vi "Convert_to_2009.vi"(8 "error in (no error)":errorcluster, 10 "2009 data in":T1={"DistSettings"={"BuildLabel"="", "ProductName"="", "BuildLocation"=path "", "MediaSize"=0, "Language"=9, "ProductVersion"={"Major"=1, "Minor"=0, "Update"=0}, "AutoIncrement"=FALSE, "ReadmeID"="", "LicenseID"="", "arpCompany"="", "arpURL"="http://", "arpContact"="", "arpPhone"="", "Executable"="", "CmdArg"="", "OSCheck"=0, "Hide"=FALSE, "LV80higher"=FALSE, "IncludeError?"=FALSE, "HWOption"=enum."<none>", "HWPath"=path "", "UpgradeCode"="", "Author"="", "MsiFileName"="", "CabFileName"="", "DistID"="", "WindowTitle"="", "WindowMessage"="", "CacheDistros"=FALSE, "EXE str ref?"=FALSE}, "BldInfo"=[], "FileInfo"=[], "DirInfo"=[], "ShortcutInfo"=[], "RegInfo"=[], "RegData"=[], "DistParts"=[], "DefaultDir"=""} {"RegData"."Values"."Type" items=["Bare", "String", "Expandable String", "Binary", "DWord"]; "DistSettings"."ProductVersion"."Update" step=1; "DistSettings"."ProductVersion"."Minor" step=1; "DistSettings"."ProductVersion"."Major" step=1; "DistSettings"."Language" items=["English"=9, "German"=7, "French"=12, "Japanese"=17, "Korean"=18, "Chinese (Simplified)"=2052]}, 11 "IB_Source_Folder in":refnum<class "IB_Source_Folder.lvclass">) -> (0 "error out":errorcluster, 2 "2009 data out":T1={"DistSettings"={"BuildLabel"="", "ProductName"="", "BuildLocation"=path "", "MediaSize"=0, "Language"=9, "ProductVersion"={"Major"=1, "Minor"=0, "Update"=0}, "AutoIncrement"=FALSE, "ReadmeID"="", "LicenseID"="", "arpCompany"="", "arpURL"="http://", "arpContact"="", "arpPhone"="", "Executable"="", "CmdArg"="", "OSCheck"=0, "Hide"=FALSE, "LV80higher"=FALSE, "IncludeError?"=FALSE, "HWOption"=enum."<none>", "HWPath"=path "", "UpgradeCode"="", "Author"="", "MsiFileName"="", "CabFileName"="", "DistID"="", "WindowTitle"="", "WindowMessage"="", "CacheDistros"=FALSE, "EXE str ref?"=FALSE}, "BldInfo"=[], "FileInfo"=[], "DirInfo"=[], "ShortcutInfo"=[], "RegInfo"=[], "RegData"=[], "DistParts"=[], "DefaultDir"=""} {"RegData"."Values"."Type" items=["Bare", "String", "Expandable String", "Binary", "DWord"]; "DistSettings"."ProductVersion"."Update" step=1; "DistSettings"."ProductVersion"."Minor" step=1; "DistSettings"."ProductVersion"."Major" step=1; "DistSettings"."Language" items=["English"=9, "German"=7, "French"=12, "Japanese"=17, "Korean"=18, "Chinese (Simplified)"=2052]})   [LabVIEW 2020, in "IB_Source_Folder.lvclass"]
uses:
  <vilib>/AppBuilder/IB_Classes/Source/Container/Folder/IB_Source_Folder.lvclass
  <vilib>/AppBuilder/IB_Classes/Source/Container/Folder/IB_Source_Folder.lvclass/IB_Source_Folder.ctl
  <vilib>/AppBuilder/IB_Classes/Source/IB_Source.lvclass
  <resource>/Framework/Providers/Builds/Installer/CDK_sTypeDef_DirInfo.ctl
  <vilib>/AppBuilder/IB_Classes/Source/Container/IB_Source_Container.lvclass
  <resource>/Framework/Providers/Builds/Installer/CDK_sTypeDef_BuildTypes.ctl
  <vilib>/AppBuilder/IB_Classes/Source/File/IB_Source_File.lvclass
  e:/builds/penguin/labview/branches/2020/dev/dist/vi.lib/AppBuilder/IB_Classes/Source/Container/IB_Source_Container.lvclass
  e:/builds/penguin/labview/branches/2020/dev/dist/vi.lib/AppBuilder/IB_Classes/Source/IB_Source.lvclass
  e:/builds/penguin/labview/branches/2020/dev/dist/vi.lib/AppBuilder/IB_Classes/Source/Container/Folder/IB_Source_Folder.lvclass
  e:/builds/penguin/labview/branches/2020/dev/dist/vi.lib/AppBuilder/IB_Classes/Source/File/IB_Source_File.lvclass
  <vilib>/AppBuilder/IB_Classes/Source/File/CtrFile/IB_CtrFile.lvclass
  e:/builds/penguin/labview/branches/2020/dev/dist/vi.lib/AppBuilder/IB_Classes/Source/File/CtrFile/IB_CtrFile.lvclass
  <resource>/Framework/Providers/Builds/Installer/CDK_sTypeDef_BuildInfo.ctl
  <resource>/Framework/Providers/Builds/Installer/CDK_sTypeDef_FileInfo.ctl
  <resource>/Framework/Providers/Builds/Installer/CDK_sTypeDef_ShortcutInfo.ctl
  <resource>/Framework/Providers/Builds/Installer/CDK_sTypeDef_Languages.ctl
  <resource>/Framework/Providers/Builds/Installer/CDK_sTypeDef_ProductVersion.ctl
  <resource>/Framework/Providers/Builds/Installer/CDK_sTypeDef_HWImportOption.ctl
  <resource>/Framework/Providers/Builds/Installer/CDK_sTypeDef_DISTSETTINGS.ctl
  AppLibs/distkit/MDF/NIMdf.llb/MDFBDPRegKeyType.ctl
  AppLibs/distkit/MDF/NI_MDF.lvlib
  <resource>/Framework/Providers/Builds/Installer/CDK_sTypeDef_RegData.ctl
  <resource>/Framework/Providers/Builds/Installer/CDK_sTypeDef_DistParts.ctl
  <vilib>/AppBuilder/IB_RW_Project/Compatibility/CDK_sTypeDef_2009_data.ctl
  <resource>/Framework/Providers/Builds/Installer/CDK_sTypeDef_SoftDep.ctl
panel:
  # "."
  # "."
  # "."
  # "."
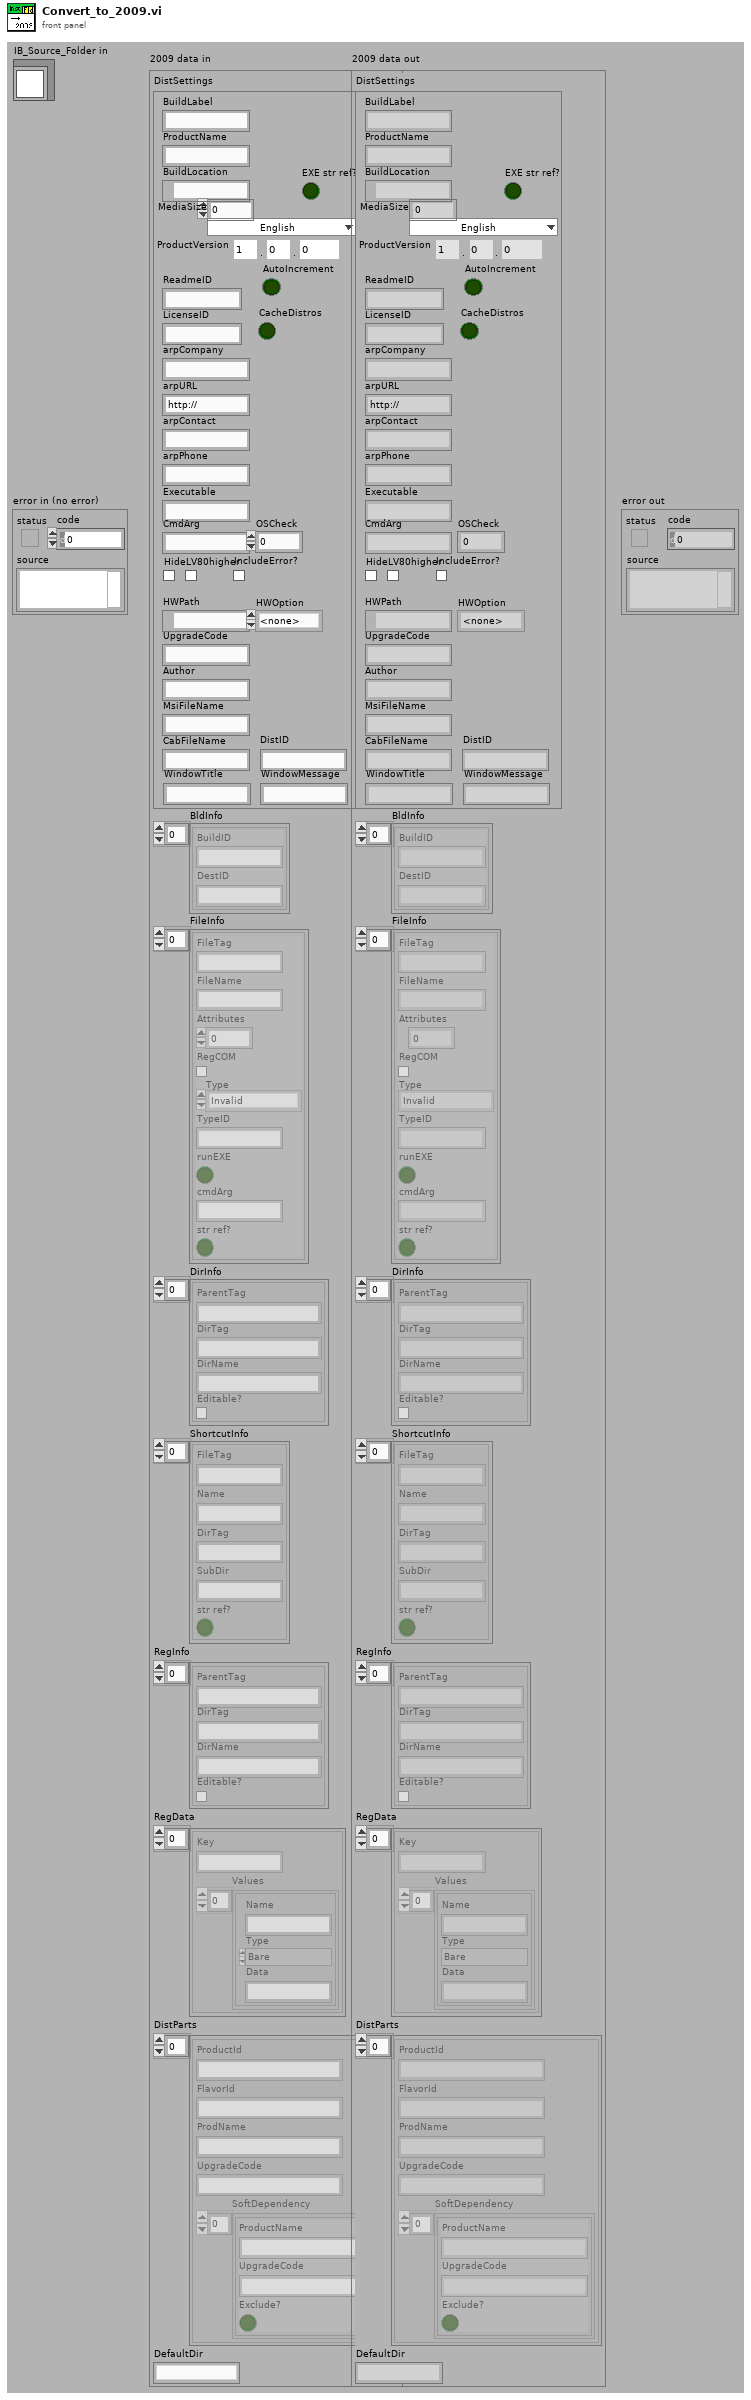
[diagram p1: front panel]
types:
  T1 = typedef "CDK_sTypeDef_2009_data.ctl" = cluster{"DistSettings":T2, "BldInfo":T6[], "FileInfo":T7[], "DirInfo":T9[], "ShortcutInfo":T10[], "RegInfo":T9[], "RegData":T11[], "DistParts":T13[], "DefaultDir":string}
  T2 = typedef "CDK_sTypeDef_DISTSETTINGS.ctl" = cluster{"BuildLabel":string, "ProductName":string, "BuildLocation":path, "MediaSize":u16, "Language":T3, "ProductVersion":T4, "AutoIncrement":bool, "ReadmeID":string, "LicenseID":string, "arpCompany":string, "arpURL":string, "arpContact":string, "arpPhone":string, "Executable":string, "CmdArg":string, "OSCheck":i32, "Hide":bool, "LV80higher":bool, "IncludeError?":bool, "HWOption":T5, "HWPath":path, "UpgradeCode":string, "Author":string, "MsiFileName":string, "CabFileName":string, "DistID":string, "WindowTitle":string, "WindowMessage":string, "CacheDistros":bool, "EXE str ref?":bool}
  T3 = typedef "CDK_sTypeDef_Languages.ctl" = u16
  T4 = typedef "CDK_sTypeDef_ProductVersion.ctl" = cluster{"Major":u8, "Minor":u8, "Update":u16}
  T5 = typedef "CDK_sTypeDef_HWImportOption.ctl" = enum16{"<none>", "Merge", "Replace", "Dialog"}
  T6 = typedef "CDK_sTypeDef_BuildInfo.ctl" = cluster{"BuildID":string, "DestID":string}
  T7 = typedef "CDK_sTypeDef_FileInfo.ctl" = cluster{"FileTag":string, "FileName":string, "Attributes":i16, "RegCOM":bool, "Type":T8, "TypeID":string, "runEXE":bool, "cmdArg":string, "str ref?":bool}
  T8 = typedef "CDK_sTypeDef_BuildTypes.ctl" = enum16{"Invalid", "File", "Folder", "BuildRule", "Library"}
  T9 = typedef "CDK_sTypeDef_DirInfo.ctl" = cluster{"ParentTag":string, "DirTag":string, "DirName":string, "Editable?":bool}
  T10 = typedef "CDK_sTypeDef_ShortcutInfo.ctl" = cluster{"FileTag":string, "Name":string, "DirTag":string, "SubDir":string, "str ref?":bool}
  T11 = typedef "CDK_sTypeDef_RegData.ctl" = cluster{"Key":string, "Values":cluster{"Name":string, "Type":T12, "Data":string}[]}
  T12 = typedef "NI_MDF.lvlib/MDFBDPRegKeyType.ctl" = i32
  T13 = typedef "CDK_sTypeDef_DistParts.ctl" = cluster{"ProductId":string, "FlavorId":string, "ProdName":string, "UpgradeCode":string, "SoftDependency":T14[]}
  T14 = typedef "CDK_sTypeDef_SoftDep.ctl" = cluster{"ProductName":string, "UpgradeCode":string, "Exclude?":bool}
  T15 = typedef "IB_Source.ctl" = cluster{"name":string, "sourceTag":string, "destTag":string, "path":path, "eng_installPath":string, "UI_inBuild?":bool, "str ref?":bool}
  T16 = typedef "IB_Source_Container.ctl" = cluster{"files":refnum<class "IB_CtrFile.lvclass">[], "previewed?":bool, "preview error?":bool}
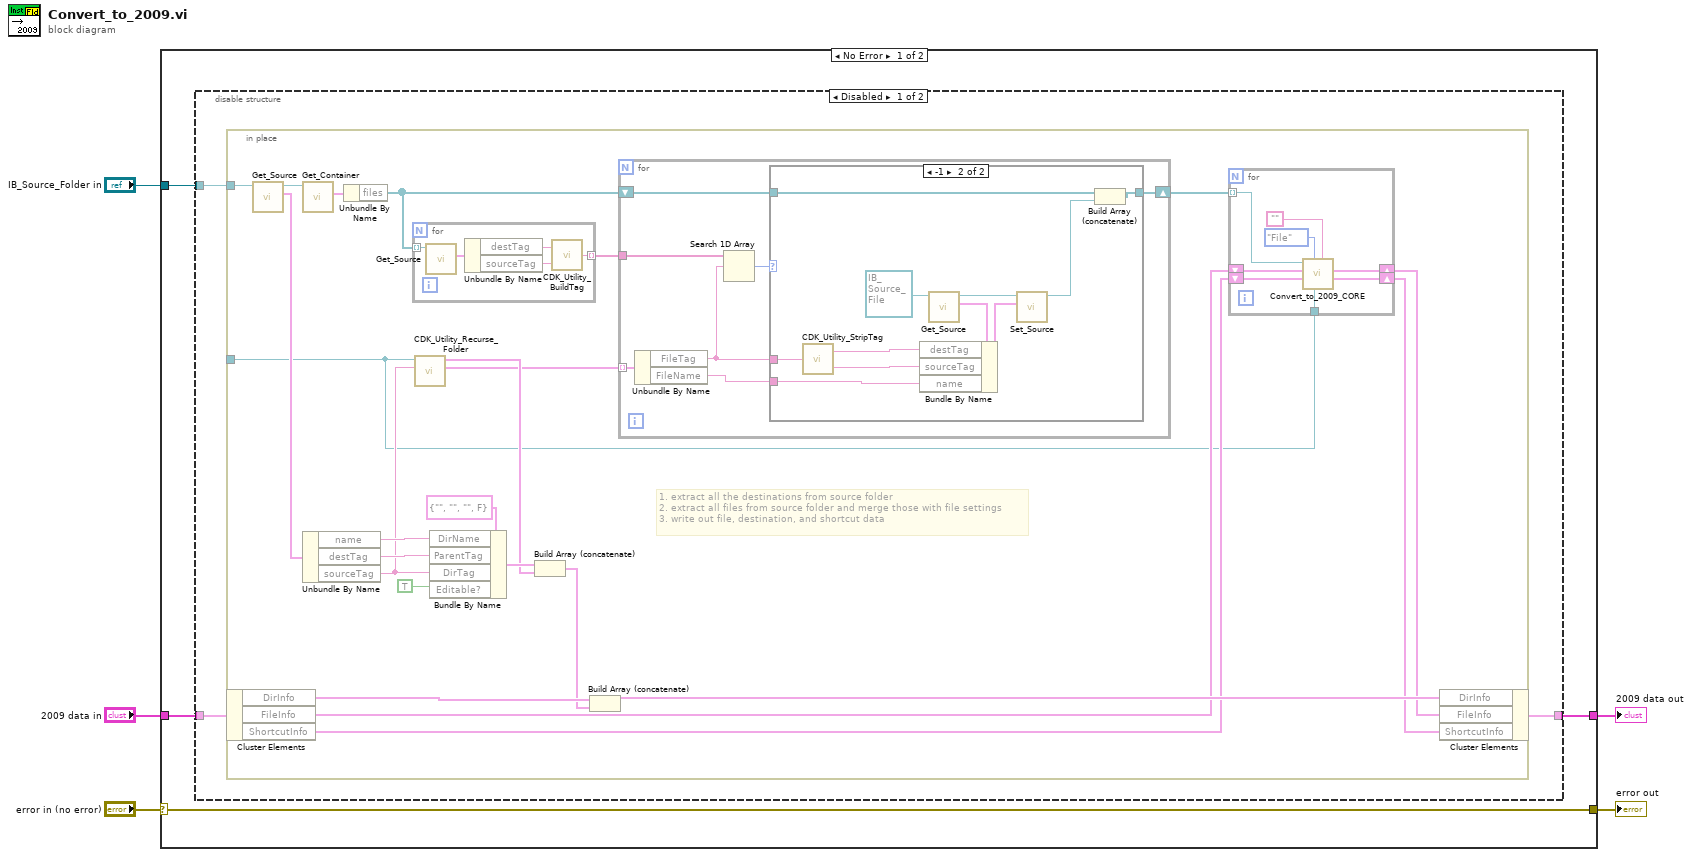
[diagram p0: block diagram]
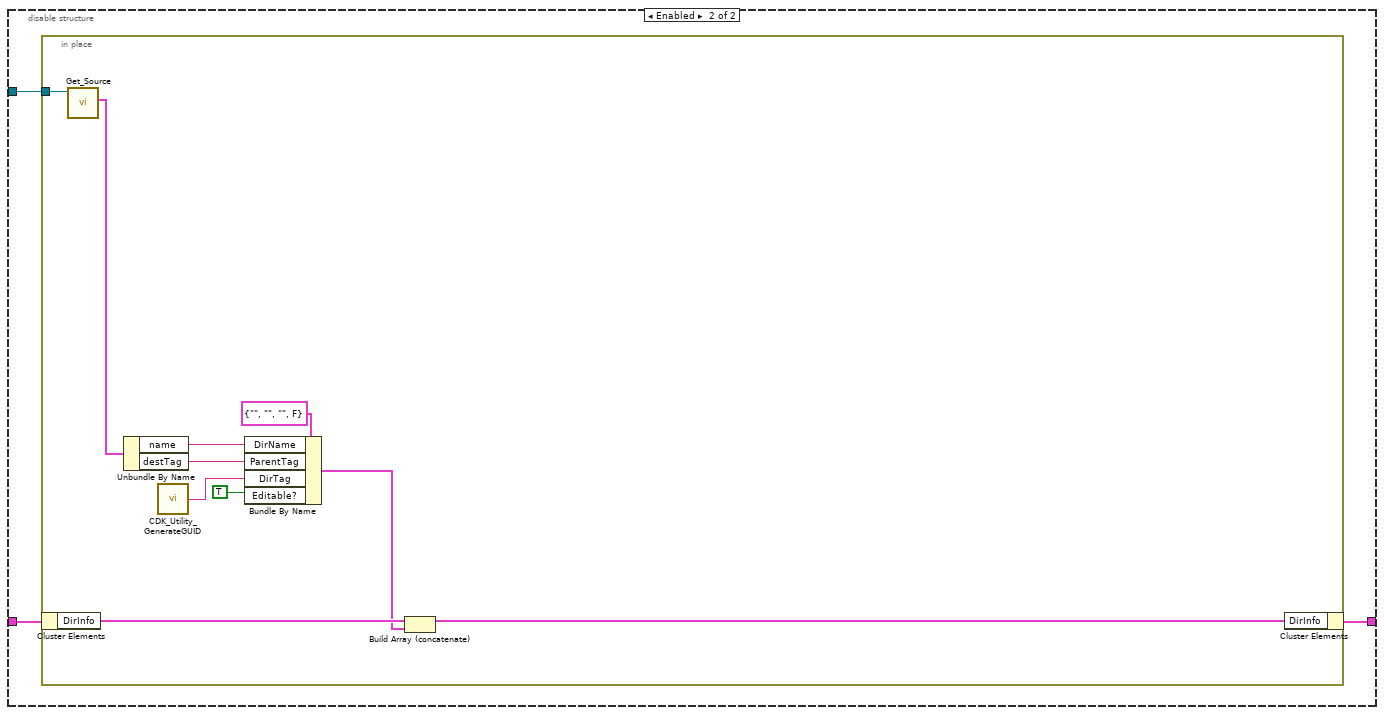
[diagram p3: hidden frame]
diagram:
  n1 = case shown="No Error" "error in (no error)" {
    selector: "error in (no error)" -> [w9 w82]
    tunnel: [w9 w82] -> w4
    tunnel: "IB_Source_Folder in" -> [w8 _]
    tunnel: "2009 data in" -> [w7 w81]
    tunnel: [w6 w81] -> w1
    frame No Error {
      n2 = disable-structure shown="Disabled" {
        disable-tunnel: w8 -> [w12 w70]
        disable-tunnel: w7 -> [w11 w69]
        disable-tunnel: [w10 w68] -> w6
        frame Disabled {
          n3 = in-place {
            in-place-border: w12 -> [w35]
            in-place-border: _ -> [w13]
            # "1. extract all the destinations from source folder\n2. extract all files from source folder and merge those with file settings\n3. write out file, destination, and shortcut data"
            n4 = in-place-cluster #1(w11) -> ("DirInfo"=w27:T9[], "FileInfo"=w20:T7[], "ShortcutInfo"=w14:T10[])
            n5 = call <vilib>:"Get_Source.vi"("IB_Source in"=w35) -> ("data"=w34:T15, "IB_Source out"=w22:refnum<class "IB_Source_Folder.lvclass">)  [unwired: 1 in, 8 out]
            n6 = call <vilib>:"Get_Container.vi"("IB_Source_Container in"=w22) -> ("data"=w23:T16)  [unwired: 1 in, 9 out]
            n7 = Unbundle By Name(w34) -> ("name"=w32:string, "destTag"=w31:string, "sourceTag"=w29:string)
            n8 = Unbundle By Name(w23) -> ("files"=w16:refnum<class "IB_CtrFile.lvclass">[])
            n9 = for {
              tunnel: w16 -> [w37] mode=indexing
              tunnel: [w36] -> w15 mode=indexing
              n10 = call <vilib>:"Get_Source.vi"("IB_Source in"=w37) -> ("data"=w38:T15)  [unwired: 1 in, 9 out]
              n11 = Unbundle By Name(w38) -> ("destTag"=w39:string, "sourceTag"=w40:string)
              n12 = call <resource>:"CDK_Utility_BuildTag.vi"("name or relative path"=w40, "BasePath"=w39) -> ("appended path"=w36:string)
            }
            n13 = call <resource>:"CDK_Utility_Recurse_Folder.vi"("sourceTag"=w29, "project ref"=w13) -> ("FileInfo out"=w17:T7[], "DirInfo out"=w28:T9[])  [unwired: 1 in, 7 out]
            n14 = Bundle By Name(cluster=T9 {"ParentTag"="", "DirTag"="", "DirName"="", "Editable?"=FALSE} ("DirInfo"), "DirName"=w32, "ParentTag"=w31, "DirTag"=w29, "Editable?"=TRUE) -> (w30:T9)
            n15 = Build Array (concatenate)(w30, w28) -> (w26:T9[])
            n16 = Build Array (concatenate)(w27, w26) -> (w25:T9[])
            n17 = for {
              tunnel: w17 -> [w44] mode=indexing
              shift-right: [w45] -> w21
              shift-left: w16 -> [w46]
              tunnel: w15 -> [w43]
              n18 = Unbundle By Name(w44) -> ("FileTag"=w42:string, "FileName"=w41:string)
              n19 = Search 1D Array(1D array=w43, element=w42) -> (index of element=w47:i32)  [unwired: 1 out]
              n20 = case shown="-1" w47 {
                tunnel: w46 -> [w48 w55]
                tunnel: [w48 w54] -> w45
                tunnel: w42 -> [_ w53]
                tunnel: w41 -> [_ w50]
                frame Default {
                  # "already found, do not add"
                }
                frame -1 {
                  n21 = call <resource>:"CDK_Utility_StripTag.vi"("Path"=w53) -> ("stripped path"=w52:string, "name"=w51:string)  [unwired: 1 in]
                  n22 = call <vilib>:"Get_Source.vi"("IB_Source in"=refnum<class "IB_Source_File.lvclass"> refnum ("IB_Source_File.lvclass")) -> ("data"=w57:T15, "IB_Source out"=w58:refnum<class "IB_Source_File.lvclass">)  [unwired: 1 in, 8 out]
                  n23 = Bundle By Name(cluster=w57, "destTag"=w52, "sourceTag"=w51, "name"=w50) -> (w56:T15)
                  n24 = call <vilib>:"Set_Source.vi"("data"=w56, "IB_Source in"=w58) -> ("IB_Source out"=w49:refnum<class "IB_Source_File.lvclass">)  [unwired: 1 in, 8 out]
                  n25 = Build Array (concatenate)(w55, w49) -> (w54:refnum<class "IB_Source_File.lvclass">[])
                }
              }
            }
            n26 = for {
              tunnel: w21 -> [w62] mode=indexing
              shift-right: [w66] -> w19
              shift-left: w20 -> [w64]
              shift-right: [w65] -> w18
              shift-left: w14 -> [w63]
              tunnel: w13 -> [w60]
              n27 = call <vilib>:"Convert_to_2009_CORE.vi"("TypeID"="", 6:w60, "Type"=CDK_sTypeDef_BuildTypes."File", "ShortcutInfoIn"=w63, "FileInfoIn"=w64, "IB_Source_File in"=w62) -> ("ShortcutInfoOut"=w65:T10[], "FileInfoOut"=w66:T7[])  [unwired: 1 in, 3 out]
            }
            n28 = in-place-cluster #1("DirInfo"=w25, "FileInfo"=w19, "ShortcutInfo"=w18) -> (w10:T1)
          }
        }
        frame Enabled {
          n29 = in-place {
            in-place-border: w70 -> [w80]
            n30 = in-place-cluster #2(w69) -> ("DirInfo"=w76:T9[])
            n31 = call <vilib>:"Get_Source.vi"("IB_Source in"=w80) -> ("data"=w73:T15)  [unwired: 1 in, 9 out]
            n32 = Unbundle By Name(w73) -> ("name"=w78:string, "destTag"=w77:string)
            n33 = call <resource>:"CDK_Utility_GenerateGUID.vi"() -> ("GUID"=w71:string)  [unwired: 9 out]
            n34 = Bundle By Name(cluster=T9 {"ParentTag"="", "DirTag"="", "DirName"="", "Editable?"=FALSE} ("DirInfo"), "DirName"=w78, "ParentTag"=w77, "DirTag"=w71, "Editable?"=TRUE) -> (w72:T9)
            n35 = Build Array (concatenate)(w76, w72) -> (w75:T9[])
            n36 = in-place-cluster #2("DirInfo"=w75) -> (w68:T1)
          }
        }
      }
    }
    frame Error {
    }
  }
  "error out" <- w4
  "2009 data out" <- w1
